vi "USBCamera2Control.vi"(2 "VideoMode":u16(ring)=5 items=["160x120 YUY2 212.22fps", "320x240 YUY2 112.49fps", "640x480 YUY2 57.84fps", "720x480 YUY2 57.84fps", "720x576 YUY2 48.43fps", "800x600 YUY2 46.53fps", "1024x768 YUY2 36.54fps", "1280x960 YUY2 29.33fps", "1600x1200 YUY2 22.53fps", "2048x1536 YUY2 18.43fps", "2590x1942 YUY2 14.61fps"], 4 "Pass":bool, 6 "Save Images Local":string, 8 "ErrorIn":errorcluster, 9 "Sequence Context In":refnum<k7>, 10 "TargetPath":path=path "C:/SNAPSHOT.BMP", 11 "Enum":T1(ring)=enum."SaveImage") -> (0 "error out":errorcluster, 1 "Image Out 1":T3(plugin-control), 3 "CamHandle":T2="cam1")   [LabVIEW 2014]
uses:
  <vilib>/userdefined/High Color/IMAQdx.ctl
  <vilib>/vision/driver/IMAQdx.llb/IMAQdx Camera Control Mode.ctl
  <vilib>/vision/driver/NI_Vision_Acquisition_Software.lvlib
  <resource>/objmgr/imaqdx.rc
panel:
  out "Init?":bool=TRUE
  out "CamSN":u32=21495273
  out "Height":u32=1942
  out "Width":u32=2590
  # "Outputs"
  # "Inputs"
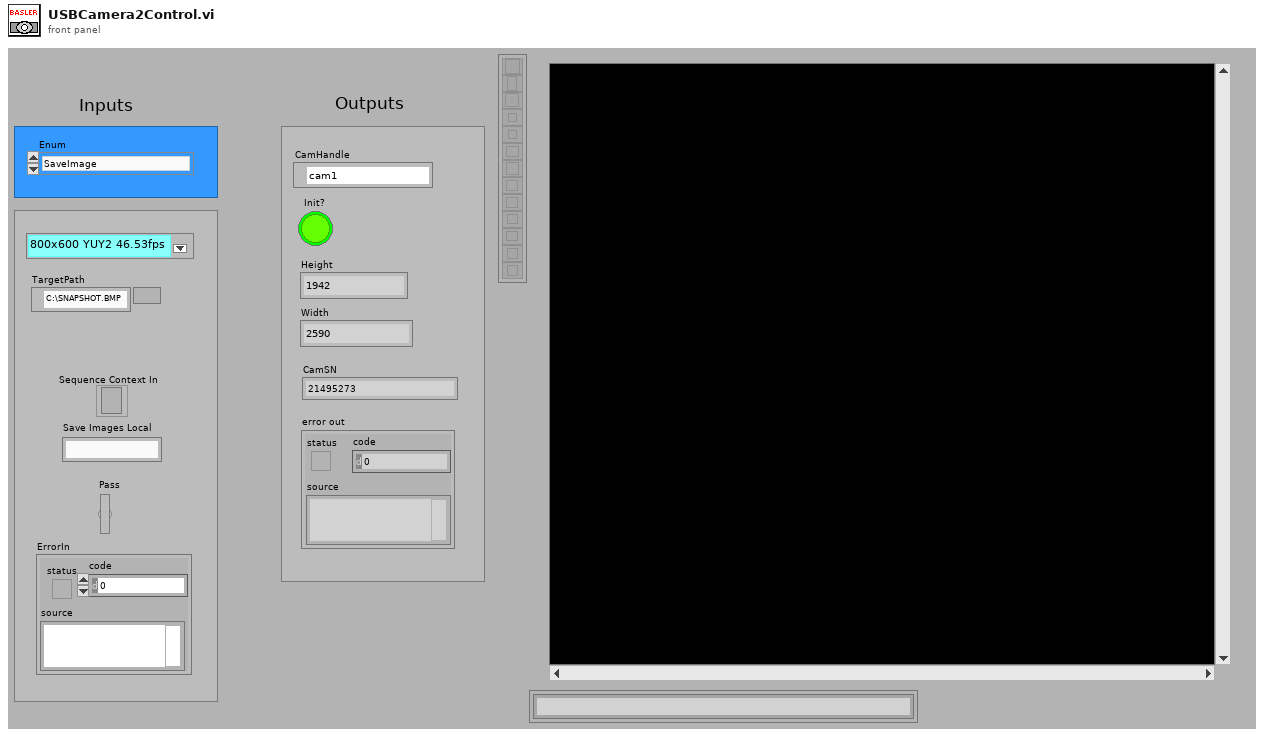
[diagram p1: front panel]
types:
  T1 = enum16{"Initialize", "Configure", "Snapshot", "SaveImage", "Close"}
  T2 = typedef "IMAQdx.ctl" = refnum<k21>
  T3 = typedef "IMAQ Image.ctl" = refnum<image>
  T4 = typedef "NI_Vision_Acquisition_Software.lvlib/IMAQdx Camera Control Mode.ctl" = enum32{"Controller", "Listener"}
  T5 = typedef "Image Type" = u32
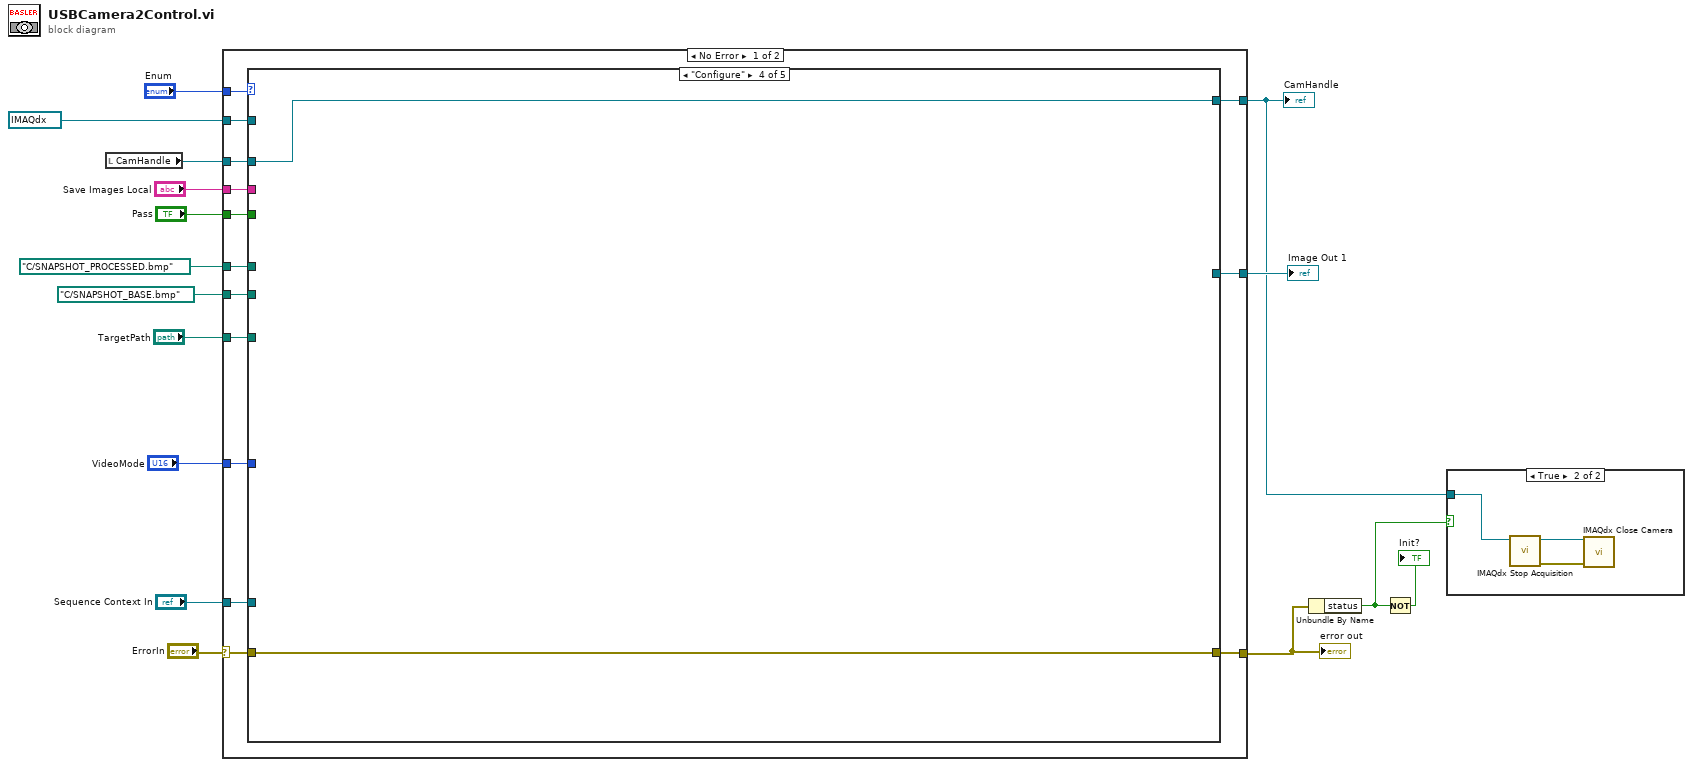
[diagram p0: block diagram]
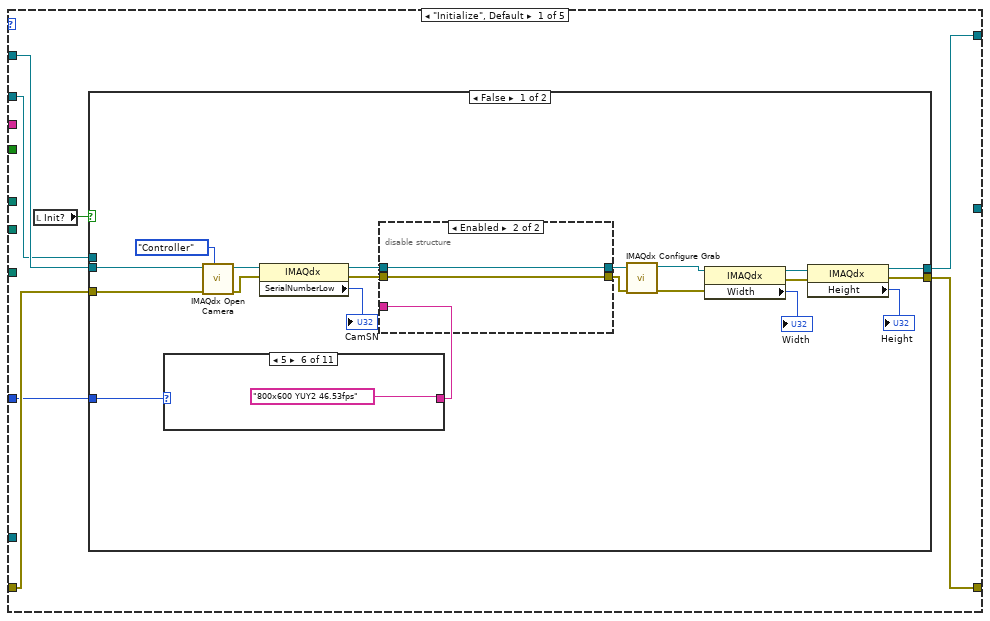
[diagram p3: hidden frame]
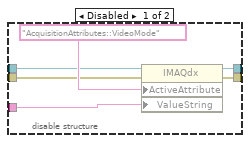
[diagram p4: hidden frame]
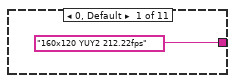
[diagram p5: hidden frame]
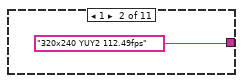
[diagram p6: hidden frame]
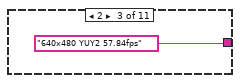
[diagram p7: hidden frame]
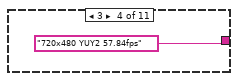
[diagram p8: hidden frame]
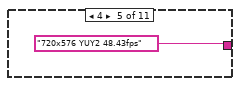
[diagram p9: hidden frame]
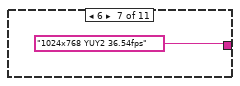
[diagram p10: hidden frame]
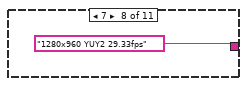
[diagram p11: hidden frame]
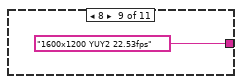
[diagram p12: hidden frame]
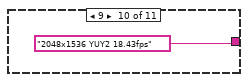
[diagram p13: hidden frame]
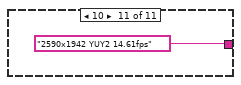
[diagram p14: hidden frame]
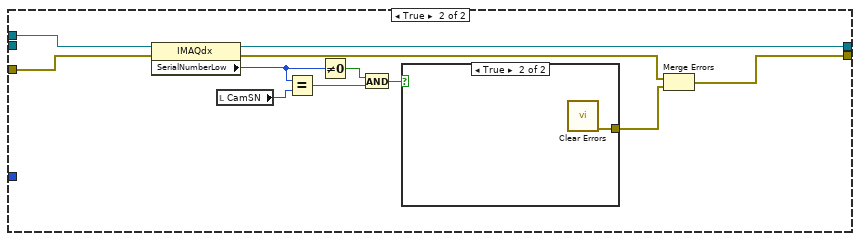
[diagram p15: hidden frame]
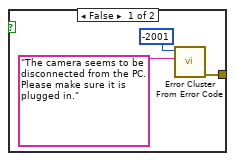
[diagram p16: hidden frame]
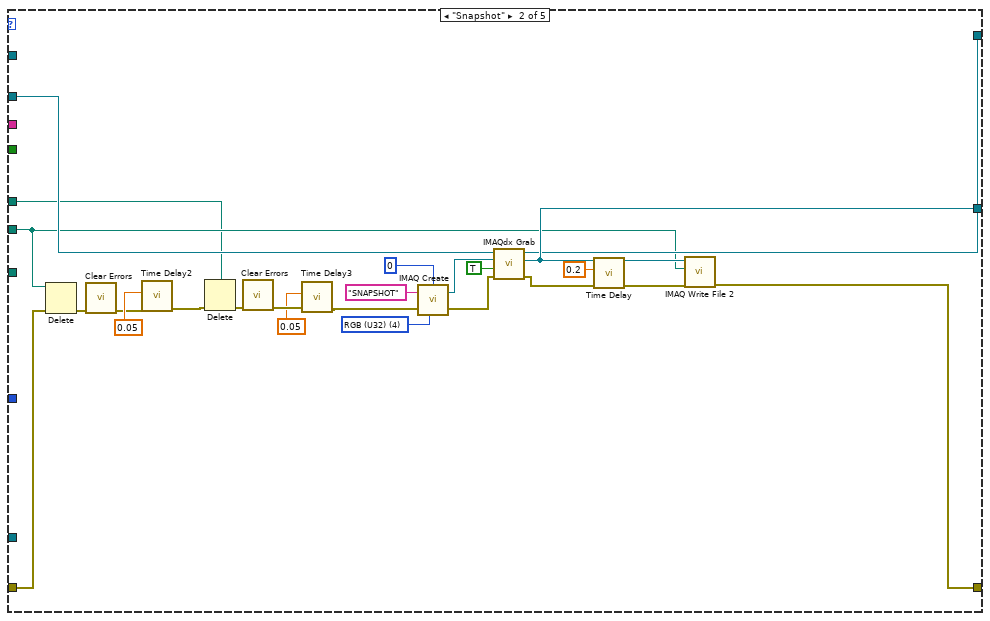
[diagram p17: hidden frame]
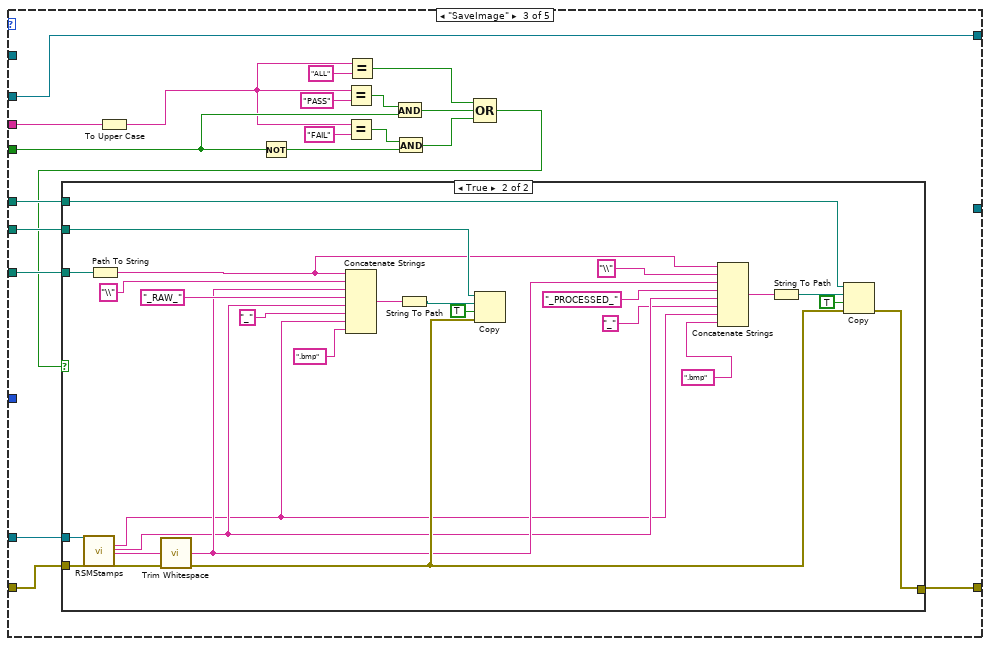
[diagram p18: hidden frame]
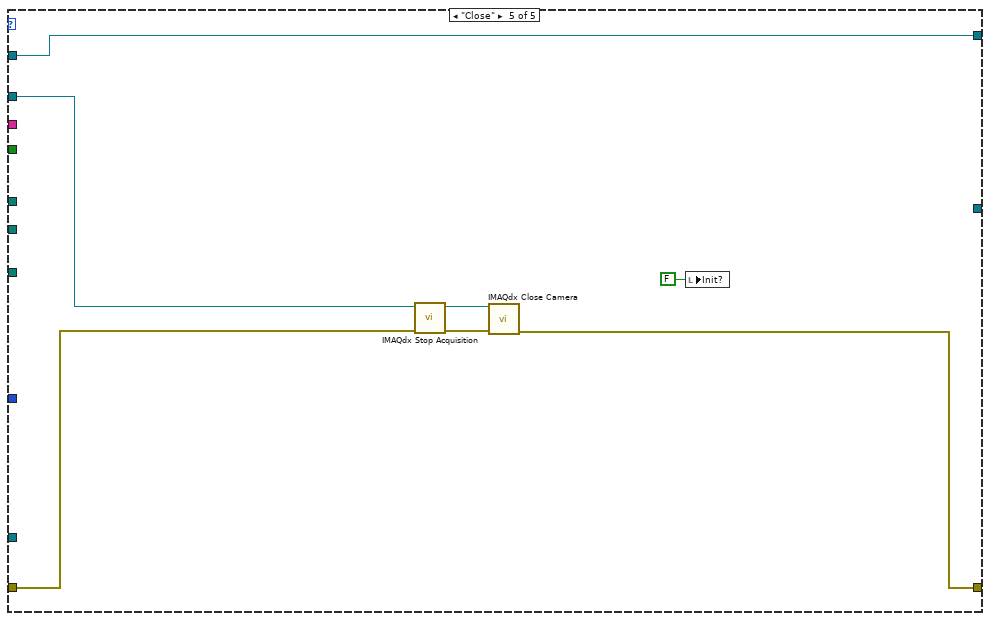
[diagram p20: hidden frame]
diagram:
  n1 = local read "CamHandle"() -> (w8:T2)
  n2 = case shown="No Error" "ErrorIn" {
    selector: "ErrorIn" -> [w28 w173]
    tunnel: [w25 w173] -> w9
    tunnel: "Enum" -> [w30 _]
    tunnel: T2 "cam1" ("Select Camera") -> [w29 w172]
    tunnel: [w27 w172] -> w1
    tunnel: w8 -> [w26 _]
    tunnel: [w24 _] -> w13
    tunnel: "TargetPath" -> [w23 _]
    tunnel: path "C:/SNAPSHOT_BASE.bmp" ("File Path") -> [w22 _]
    tunnel: "VideoMode" -> [w21 _]
    tunnel: path "C:/SNAPSHOT_PROCESSED.bmp" ("File Path") -> [w20 _]
    tunnel: "Sequence Context In" -> [w18 _]
    tunnel: "Save Images Local" -> [w19 _]
    tunnel: "Pass" -> [w17 _]
    frame No Error {
      n3 = case shown="\"Configure\"" w30 {
        tunnel: w29 -> [w36 _ _ _ w166]
        tunnel: w28 -> [w37 w105 w129 w164 w168]
        tunnel: [w31 w106 w134 w163 w166] -> w27
        tunnel: [w35 w109 w132 w164 w167] -> w25
        tunnel: w26 -> [w33 w111 w134 w163 w169]
        tunnel: [_ w108 _ _ _] -> w24
        tunnel: w23 -> [_ _ w135 _ _]
        tunnel: w22 -> [_ w104 w133 _ _]
        tunnel: w21 -> [w32 _ _ _ _]
        tunnel: w20 -> [_ w98 w131 _ _]
        tunnel: w19 -> [_ _ w124 _ _]
        tunnel: w18 -> [_ _ w130 _ _]
        tunnel: w17 -> [_ _ w125 _ _]
        frame "Initialize", Default {
          n4 = local read "Init?"() -> (w34:bool)
          n5 = case shown="False" w34 {
            tunnel: w37 -> [w52 w86]
            tunnel: w36 -> [w51 _]
            tunnel: [w45 w85] -> w31
            tunnel: [w44 w77] -> w35
            tunnel: w33 -> [_ w87]
            tunnel: w32 -> [w39 _]
            frame False {
              n6 = case shown="5" w39 {
                tunnel: ["160x120 YUY2 212.22fps" ("ValueString") "320x240 YUY2 112.49fps" ("ValueString") "640x480 YUY2 57.84fps" ("ValueString") "720x480 YUY2 57.84fps" ("ValueString") "720x576 YUY2 48.43fps" ("ValueString") "800x600 YUY2 46.53fps" ("ValueString") "1024x768 YUY2 36.54fps" ("ValueString") "1280x960 YUY2 29.33fps" ("ValueString") "1600x1200 YUY2 22.53fps" ("ValueString") "2048x1536 YUY2 18.43fps" ("ValueString") "2590x1942 YUY2 14.61fps" ("ValueString")] -> w38
                frame 0, Default {
                }
                frame 1 {
                }
                frame 2 {
                }
                frame 3 {
                }
                frame 4 {
                }
                frame 5 {
                }
                frame 6 {
                }
                frame 7 {
                }
                frame 8 {
                }
                frame 9 {
                }
                frame 10 {
                }
              }
              n7 = call <vilib>:"IMAQdx Open Camera.vi"("Camera Control Mode"=IMAQdx_Camera_Control_Mode."Controller", "error in"=w52, "Session In"=w51) -> ("error out"=w49:errorcluster, "Session Out"=w50:T2)  [unwired: 7 in]
              n8 = property class="IMAQdx"(reference=w50, error in=w49) -> (reference out=w43:T2, error out=w42:errorcluster, "SerialNumberLow"=→"CamSN":u32)
              n9 = disable-structure shown="Enabled" {
                disable-tunnel: w43 -> [w62 w65]
                disable-tunnel: w42 -> [w61 w64]
                disable-tunnel: [w60 w65] -> w41
                disable-tunnel: [w59 w64] -> w40
                disable-tunnel: w38 -> [w58 _]
                frame Disabled {
                  n10 = property class="IMAQdx"(reference=w62, error in=w61, "ActiveAttribute"="AcquisitionAttributes::VideoMode", "ValueString"=w58) -> (reference out=w60:T2, error out=w59:errorcluster)
                }
                frame Enabled {
                }
              }
              n11 = call <vilib>:"IMAQdx Configure Grab.vi"("error in"=w40, "Session In"=w41) -> ("error out"=w54:errorcluster, "Session Out"=w53:T2)  [unwired: 8 in]
              n12 = property class="IMAQdx"(reference=w53, error in=w54) -> (reference out=w55:T2, error out=w56:errorcluster, "Width"=→"Width":u32)
              n13 = property class="IMAQdx"(reference=w55, error in=w56) -> (reference out=w45:T2, error out=w44:errorcluster, "Height"=→"Height":u32)
            }
            frame True {
              n14 = property class="IMAQdx"(reference=w87, error in=w86) -> (reference out=w85:T2, error out=w78:errorcluster, "SerialNumberLow"=w83:u32)
              n15 = local read "CamSN"() -> (w84:u32)
              n16 = Equal?(x=w83, y=w84) -> (x = y?=w81:bool)
              n17 = Not Equal To 0?(x=w83) -> (x != 0?=w82:bool)
              n18 = And(x=w82, y=w81) -> (x .and. y?=w80:bool)
              n19 = case shown="True" w80 {
                tunnel: [w89 w91] -> w79
                frame False {
                  n20 = call <vilib>:"Error Cluster From Error Code.vi"("error message (\"\")"="The camera seems to be disconnected from the PC. Please make sure it is plugged in." ("error message (\"\")"), "error code (0)"=-2001) -> ("error out"=w89:errorcluster)  [unwired: 7 in]
                }
                frame True {
                  n21 = call <vilib>:"Clear Errors.vi"() -> ("error out"=w91:errorcluster)  [unwired: 6 in, 1 out]
                }
              }
              n22 = Merge Errors(w78, w79) -> (w77:errorcluster)
            }
          }
        }
        frame "Snapshot" {
          w114 = T5 4 items=["Grayscale (U8)", "Grayscale (I16)", "Grayscale (SGL)", "Complex (CSG)", "RGB (U32)", "HSL (U32)", "RGB (U64)", "Grayscale (U16)"] ("Image Type")
          n23 = Delete(path (use dialog)=w104, error in=w105) -> (error out=w99:errorcluster)  [unwired: 3 in, 2 out]
          n24 = call <vilib>:"Clear Errors.vi"("error in (no error)"=w99) -> ("error out"=w96:errorcluster)  [unwired: 5 in, 1 out]
          n25 = call "Time Delay2"("error in (no error)"=w96, "Delay Time (s)"=0.05) -> ("error out"=w95:errorcluster)  [unwired: 9 in]
          n26 = Delete(path (use dialog)=w98, error in=w95) -> (error out=w100:errorcluster)  [unwired: 3 in, 2 out]
          n27 = call <vilib>:"Clear Errors.vi"("error in (no error)"=w100) -> ("error out"=w94:errorcluster)  [unwired: 5 in, 1 out]
          n28 = call "Time Delay3"("error in (no error)"=w94, "Delay Time (s)"=0.05) -> ("error out"=w93:errorcluster)  [unwired: 9 in]
          n29 = call "IMAQ Create"("Border Size"=0, "Image Name"="SNAPSHOT", "Image Type"=w114, "error in (no error)"=w93) -> ("New Image"=w112:T3, "error out"=w110:errorcluster)  [unwired: 1 in]
          n30 = call <vilib>:"IMAQdx Grab.vi"("error in"=w110, "Wait for Next Buffer? (Yes)"=TRUE, "Image In"=w112, "Session In"=w111) -> ("error out"=w103:errorcluster, "Image Out"=w108:T3, "Session Out"=w106:T2)  [unwired: 4 in, 1 out]
          n31 = call "Time Delay"("error in (no error)"=w103, "Delay Time (s)"=0.2) -> ("error out"=w102:errorcluster)  [unwired: 9 in]
          n32 = call-poly "IMAQ Write File 2"("error in (no error)"=w102, "File Path"=w104, "Image"=w108) -> ("error out"=w109:errorcluster)  [unwired: 7 in, 1 out]
        }
        frame "SaveImage" {
          n33 = To Upper Case(1:w124) -> (0:w122:string)
          n34 = Not(x=w125) -> (.not. x?=w121:bool)
          n35 = Equal?(x=w122, y="PASS") -> (x = y?=w126:bool)
          n36 = Equal?(x=w122, y="FAIL") -> (x = y?=w120:bool)
          n37 = Equal?(x=w122, y="ALL") -> (x = y?=w118:bool)
          n38 = And(x=w126, y=w125) -> (x .and. y?=w119:bool)
          n39 = And(x=w120, y=w121) -> (x .and. y?=w117:bool)
          n40 = Compound Arithmetic op=OR(w118, w119, w117) -> (w116:bool)
          n41 = case shown="True" w116 {
            tunnel: w135 -> [_ w161]
            tunnel: w133 -> [_ w159]
            tunnel: [w136 w157] -> w132
            tunnel: w131 -> [_ w156]
            tunnel: w130 -> [_ w153]
            tunnel: w129 -> [w136 w150]
            frame False {
            }
            frame True {
              n42 = call "RSMStamps.vi"("Sequence Context In"=w153, "error IN"=w150) -> ("TimeStamp"=w138:string, "DateStamp"=w140:string, "SerialNumber"=w151:string, "error Out"=w143:errorcluster)  [unwired: 19 in, 3 out]
              n43 = Path To String(path=w161) -> (string=w145:string)
              n44 = call <vilib>:"Trim Whitespace.vi"("string"=w151) -> ("trimmed string"=w142:string)  [unwired: 1 in]
              n45 = Concatenate Strings(w145, "\\" ("string"), w142, "_RAW_" ("string"), w140, "_" ("string"), w138, ".bmp" ("string")) -> (w146:string)
              n46 = String To Path(string=w146) -> (path=w152:path)
              n47 = Copy(8:w143, 9:TRUE ("overwrite (F)"), 10:w152, 11:w159) -> ()  [unwired: 1 in, 3 out]
              n48 = Concatenate Strings(w145, "\\" ("string"), w142, "_PROCESSED_" ("string"), w140, "_" ("string"), w138, ".bmp" ("string")) -> (w155:string)
              n49 = String To Path(string=w155) -> (path=w154:path)
              n50 = Copy(8:w143, 9:TRUE ("overwrite (F)"), 10:w154, 11:w156) -> (0:w157:errorcluster)  [unwired: 1 in, 2 out]
            }
          }
        }
        frame "Configure" {
        }
        frame "Close" {
          n51 = call <vilib>:"IMAQdx Stop Acquisition.vi"("error in"=w168, "Session In"=w169) -> ("error out"=w171:errorcluster, "Session Out"=w170:T2)  [unwired: 8 in]
          n52 = call <vilib>:"IMAQdx Close Camera.vi"("error in"=w171, "Session In"=w170) -> ("error out"=w167:errorcluster)  [unwired: 9 in]
          n53 = local write "Init?"(FALSE ("Init?")) -> ()
        }
      }
    }
    frame Error {
    }
  }
  "error out" <- w9
  "CamHandle" <- w1
  "Image Out 1" <- w13
  n54 = Unbundle By Name(w9) -> ("status"=w2:bool)
  n55 = Not(x=w2) -> (.not. x?=→"Init?":bool)
  n56 = case shown="True" w2 {
    tunnel: w1 -> [_ w174]
    frame False {
    }
    frame True {
      n57 = call <vilib>:"IMAQdx Stop Acquisition.vi"("Session In"=w174) -> ("error out"=w176:errorcluster, "Session Out"=w175:T2)  [unwired: 9 in]
      n58 = call <vilib>:"IMAQdx Close Camera.vi"("error in"=w176, "Session In"=w175) -> ()  [unwired: 9 in, 1 out]
    }
  }
